vi "FSK_Demodulation.vi"(0 "PathIn":path, 2 "input_data":cdb[](array[numeric]), 7 "FreqCarrier1":dbl format="%#_13g", 9 "FreqCarrier2":dbl format="%#_13g", 11 "error in (no error)":errorcluster caption="错误输入（无错误）") -> (4 "PathOut":path, 6 "RecvFskDemod":cdb[](array[numeric]) format="%#_13g", 15 "error out":errorcluster caption="错误输出")   [LabVIEW 2015]
panel:
  out "SendSig1 2":dbl[](array[numeric]) format="%#_13g"
  out "SendSig1":dbl[](array[numeric]) format="%#_13g"
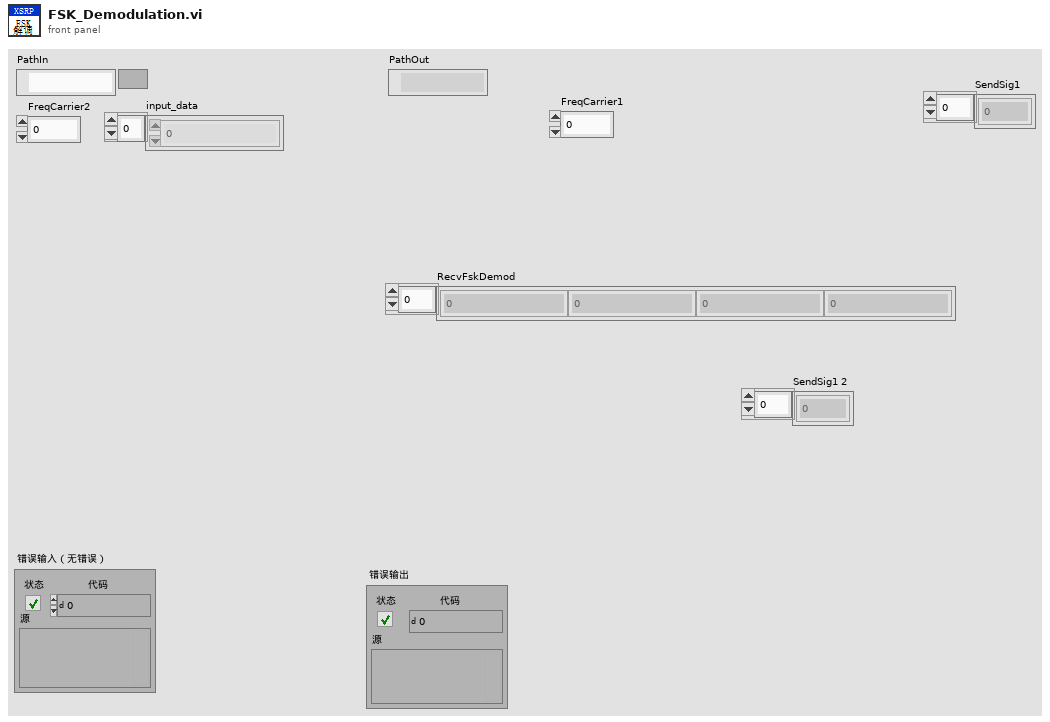
[diagram p1: front panel]
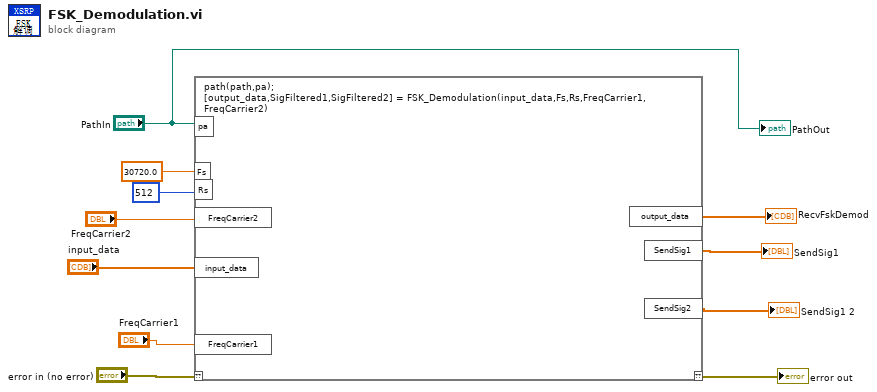
[diagram p0: block diagram]
diagram:
  n1 = script code="path(path,pa);\n[output_data,SigFiltered1,SigFiltered2] = FSK_Demodulation(input_data,Fs,Rs,FreqCarrier1, FreqCarrier2)"("??"="error in (no error)", "pa"="PathIn", "input_data"="input_data", "Fs"=30720.0, "FreqCarrier1"="FreqCarrier1", "FreqCarrier2"="FreqCarrier2", "Rs"=512) -> ("??"=→"error out":errorcluster, "output_data"=→"RecvFskDemod":cdb[], "SendSig1"=→"SendSig1":dbl[], "SendSig2"=→"SendSig1 2":dbl[])
  "PathOut" <- "PathIn"
